vi "ADInfo.vi"(0 "refnum":refnum<file>, 11 "offset":i32) -> (2 "A/D info":T1={"# rf points per line"=0, "# lines per scan"=0, "sample rate MHz"=0, "# A/D bits"=8, "# bytes per A/D"=1, "TGC Flag"=0, "A/D Type"=""}, 4 "dup refnum":refnum<file>, 6 "# rf points per line":u16, 8 "# lines per scan":u16, 10 "sample rate MHz":u16, 12 "A/D Type":string, 13 "TGC Flag":u16, 14 "# bytes per A/D":u16, 15 "# A/D bits":u16)   [LabVIEW 2022 SP3]
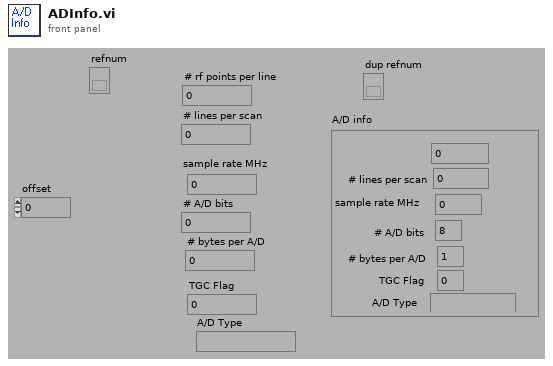
[diagram p1: front panel]
types:
  T1 = cluster{"# rf points per line":u16, "# lines per scan":u16, "sample rate MHz":u16, "# A/D bits":i16, "# bytes per A/D":u16, "TGC Flag":u16, "A/D Type":string}
  T2 = enum16{"big-endian, network order", "native, host order", "little-endian"}
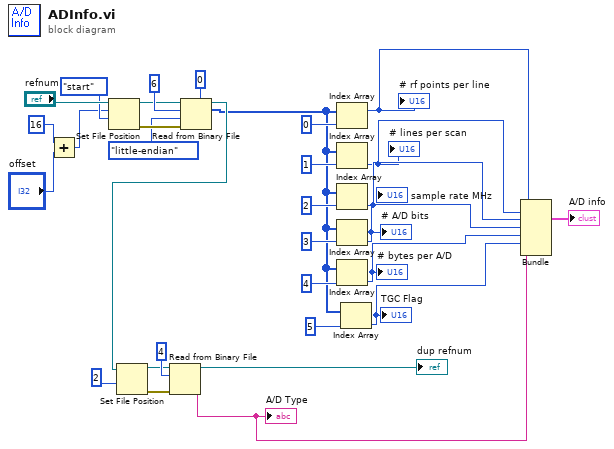
[diagram p0: block diagram]
diagram:
  n1 = Add(x=16 ("pos offset (0)"), y="offset") -> (x+y=w7:i32)
  n2 = Set File Position(offset (in bytes) (0)=w7, refnum="refnum", from (0:start)=enum16{"start", "end", "current"}."start" ("pos mode (0:2)")) -> (refnum out=w4:refnum<file>, error out=w3:errorcluster)  [unwired: 1 in]
  n3 = Read from Binary File(5:u16 0, 8:w3, 9:T2."little-endian" ("byte order (0:big-endian, network order)"), 10:6 ("count"), 11:w4) -> (2:w2:u16[], 3:w24:refnum<file>)  [unwired: 3 out]
  n4 = Set File Position(refnum=w24, from (0:start)=2) -> (refnum out=w6:refnum<file>, error out=w5:errorcluster)  [unwired: 1 in, 1 out]
  n5 = Read from Binary File(8:w5, 10:4 ("count"), 11:w6) -> (2:w17:string, 3:→"dup refnum":refnum<file>)  [unwired: 5 out]
  "A/D Type" <- w17
  n6 = Index Array(array=w2, index=0) -> (element=w11:u16)
  "# rf points per line" <- w11
  n7 = Index Array(array=w2, index=1) -> (element=w12:u16)
  "# lines per scan" <- w12
  n8 = Index Array(array=w2, index=2) -> (element=w13:u16)
  "sample rate MHz" <- w13
  n9 = Index Array(array=w2, index=3) -> (element=w14:u16)
  "# A/D bits" <- w14
  n10 = Index Array(array=w2, index=4) -> (element=w15:u16)
  "# bytes per A/D" <- w15
  n11 = Index Array(array=w2, index=5) -> (element=w16:u16)
  "TGC Flag" <- w16
  n12 = Bundle(w11, w12, w13, w14, w15, w16, w17) -> (→"A/D info":cluster{u16, u16, u16, u16, u16, u16, string})  [unwired: 1 out]
